vi "Write Kierunek.vi"(8 "error in (no error)":errorcluster, 10 "Kierunek":i16, 11 "Boid in":refnum<class "Boid.lvclass">) -> (0 "error out":errorcluster, 3 "Boid out":refnum<class "Boid.lvclass">)   [LabVIEW 2014, in "Boid.lvclass"]
uses:
  Boid.lvclass
  Boid.lvclass/Boid.ctl
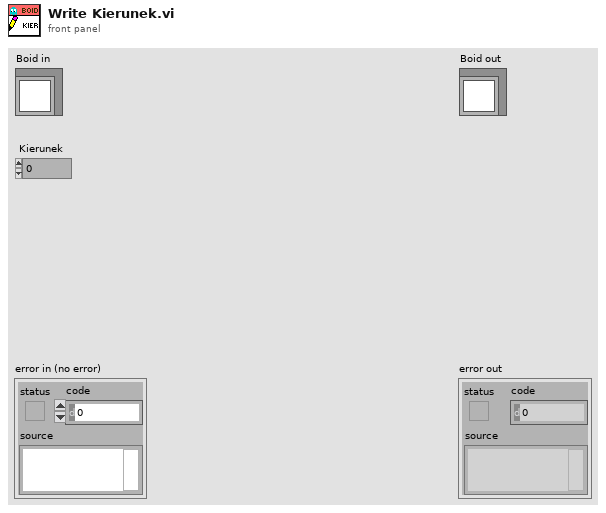
[diagram p1: front panel]
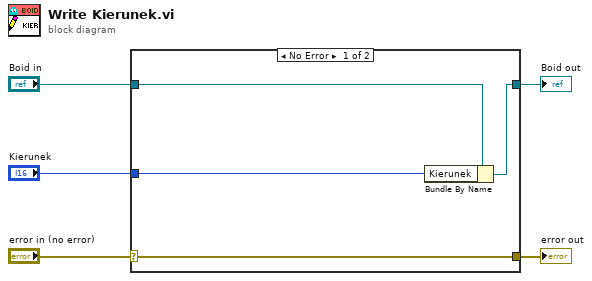
[diagram p0: block diagram]
diagram:
  n1 = case shown="No Error" "error in (no error)" {
    selector: "error in (no error)" -> [w9 w10]
    tunnel: [w9 w10] -> w4
    tunnel: [w7 w11] -> w2
    tunnel: "Boid in" -> [w8 w11]
    tunnel: "Kierunek" -> [w6 _]
    frame No Error {
      n2 = Bundle By Name(cluster=w8, "Kierunek"=w6) -> (w7:refnum<class "Boid.lvclass">)
    }
    frame Error {
    }
  }
  "error out" <- w4
  "Boid out" <- w2
